vi "Read Associated Controller Actor Enqueuer.vi"(8 "error in (no error)":errorcluster, 11 "CS++GUIActor in":refnum<class "CS++GUIActor.lvclass">) -> (0 "error out":errorcluster, 2 "Actor Framework:Message Enqueuer":refnum<class "Message Enqueuer.lvclass">, 3 "CS++GUIActor out":refnum<class "CS++GUIActor.lvclass">)   [LabVIEW 2014, in "CS++GUIActor.lvlib" / "CS++GUIActor.lvclass"]
uses:
  CS++GUIActor.lvclass
  <vilib>/ActorFramework/Message Enqueuer/Message Enqueuer.lvclass
  CS++GUIActor.lvclass/CS++GUIActor.ctl
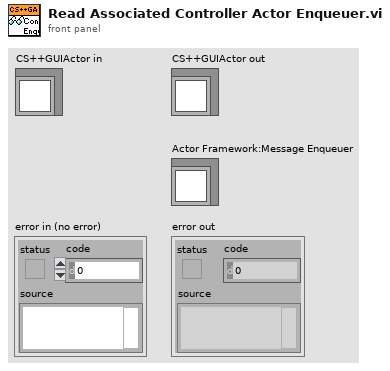
[diagram p1: front panel]
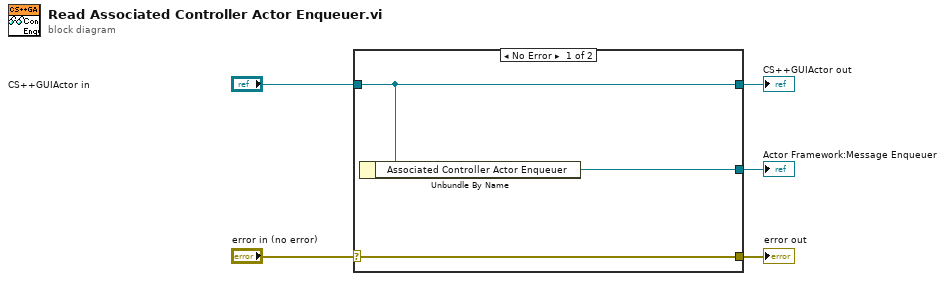
[diagram p0: block diagram]
diagram:
  n1 = case shown="No Error" "error in (no error)" {
    selector: "error in (no error)" -> [w8 w9]
    tunnel: [w8 w9] -> w4
    tunnel: [w7 w10] -> w2
    tunnel: "CS++GUIActor in" -> [w7 w10]
    tunnel: [w6 _] -> w1
    frame No Error {
      n2 = Unbundle By Name(w7) -> ("Associated Controller Actor Enqueuer"=w6:refnum<class "Message Enqueuer.lvclass">)
    }
    frame Error {
    }
  }
  "error out" <- w4
  "CS++GUIActor out" <- w2
  "Actor Framework:Message Enqueuer" <- w1
